vi "Changed Value Pair.vi"(8 "error in (no error)":errorcluster, 10 "Value Pairs":T1, 11 "Boolean Data Type in":refnum<class "Boolean Data Type.lvclass">) -> (0 "error out":errorcluster, 3 "Boolean Data Type out":refnum<class "Boolean Data Type.lvclass">)   [LabVIEW 2018, in "Boolean Data Type.lvclass"]
uses:
  Boolean Data Type.lvclass
  Value Pairs.ctl
  Boolean Data Type.lvclass/Boolean Data Type.ctl
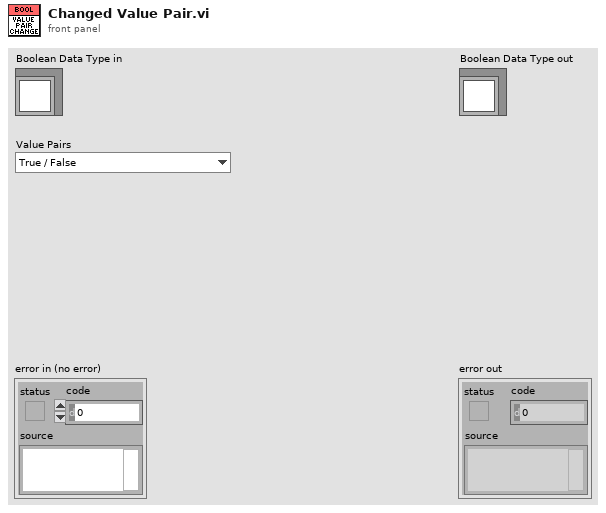
[diagram p1: front panel]
types:
  T1 = typedef "Boolean Data Type.lvclass/Value Pairs.ctl" = enum16{"True / False", "Yes / No", "X / [Blank]", "On / Off", "Custom"}
  T2 = enum8{"Enabled", "Disabled", "Disabled and Grayed Out"}
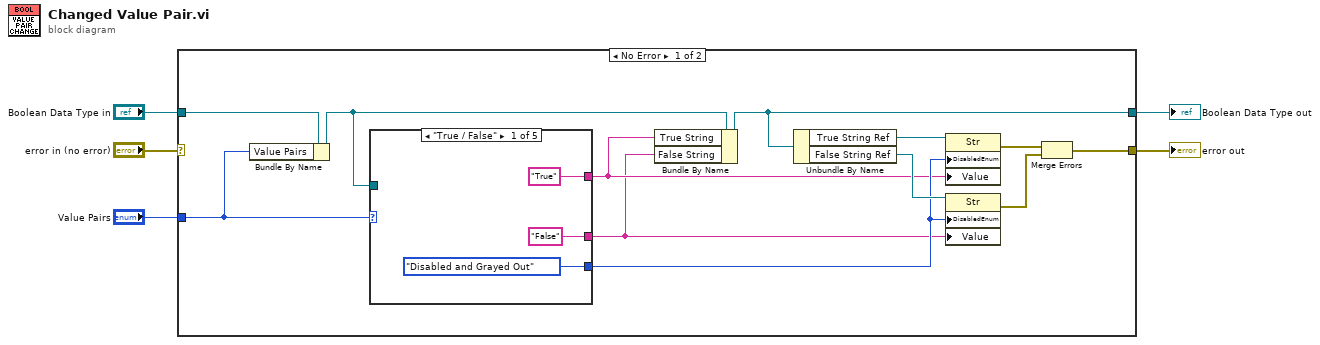
[diagram p0: block diagram]
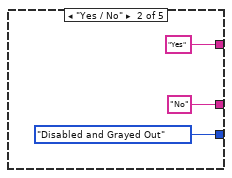
[diagram p2: hidden frame]
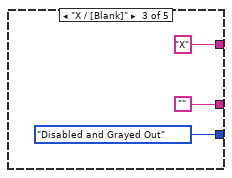
[diagram p3: hidden frame]
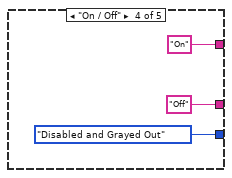
[diagram p4: hidden frame]
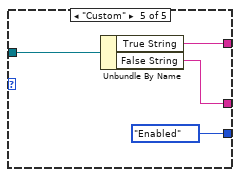
[diagram p5: hidden frame]
diagram:
  n1 = case shown="No Error" "error in (no error)" {
    selector: "error in (no error)" -> [_ w35]
    tunnel: [w12 w35] -> w4
    tunnel: [w8 w34] -> w2
    tunnel: "Boolean Data Type in" -> [w10 w34]
    tunnel: "Value Pairs" -> [w11 _]
    frame No Error {
      n2 = Bundle By Name(cluster=w10, "Value Pairs"=w11) -> (w9:refnum<class "Boolean Data Type.lvclass">)
      n3 = case shown="\"True / False\"" w11 {
        tunnel: [T2."Disabled and Grayed Out" ("Disabled") T2."Disabled and Grayed Out" ("Disabled") T2."Disabled and Grayed Out" ("Disabled") T2."Disabled and Grayed Out" ("Disabled") T2."Enabled" ("Disabled")] -> w15
        tunnel: ["True" "Yes" "X" "On" w31] -> w7
        tunnel: ["False" "No" "" "Off" w30] -> w6
        tunnel: w9 -> [_ _ _ _ w32]
        frame "True / False" {
        }
        frame "Yes / No" {
        }
        frame "X / [Blank]" {
        }
        frame "On / Off" {
        }
        frame "Custom" {
          n4 = Unbundle By Name(w32) -> ("True String"=w31:string, "False String"=w30:string)
        }
      }
      n5 = Bundle By Name(cluster=w9, "True String"=w7, "False String"=w6) -> (w8:refnum<class "Boolean Data Type.lvclass">)
      n6 = Unbundle By Name(w8) -> ("True String Ref"=w17:refnum<vi>, "False String Ref"=w16:refnum<vi>)
      n7 = property class="Str"(reference=w17, "DisabledEnum"=w15, "Value"=w7) -> (error out=w14:errorcluster)  [unwired: 1 in, 1 out]
      n8 = property class="Str"(reference=w16, "DisabledEnum"=w15, "Value"=w6) -> (error out=w13:errorcluster)  [unwired: 1 in, 1 out]
      n9 = Merge Errors(w14, w13) -> (w12:errorcluster)
    }
    frame Error {
    }
  }
  "error out" <- w4
  "Boolean Data Type out" <- w2
